vi "获取需发送的数据表.vi"(8 "error in (no error)":errorcluster) -> (0 "error out":errorcluster, 3 "tables":string[](array[string]))   [LabVIEW 2016, in "数据传输系统-03.lvlib"]
uses:
  <vilib>/Utility/sysdir.llb/System Directory Type.ctl
  <vilib>/addons/database/Connection.llb/DB Tools Open Connec (String).vi
  <vilib>/addons/database/NI_Database_API.lvlib
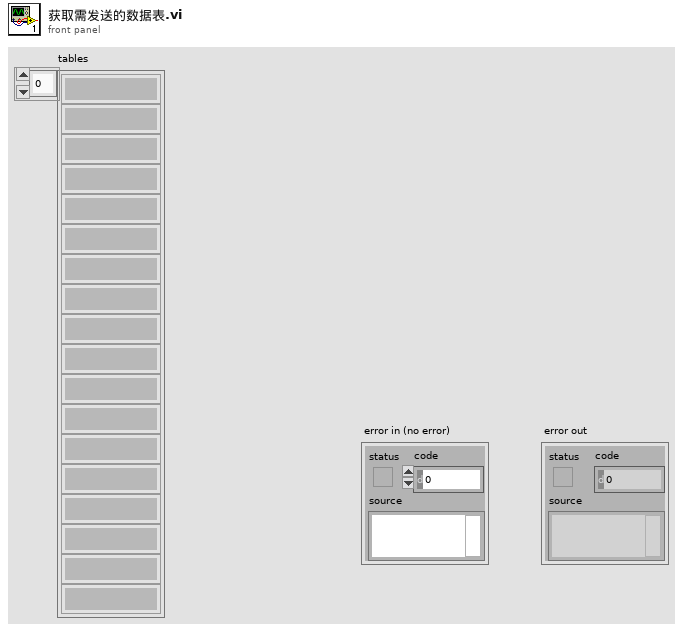
[diagram p1: front panel]
types:
  T1 = typedef "System Directory Type.ctl" = i32
  T2 = typedef "NI_Database_API.lvlib/Conn ObjectReference.ctl" = refnum<k1>
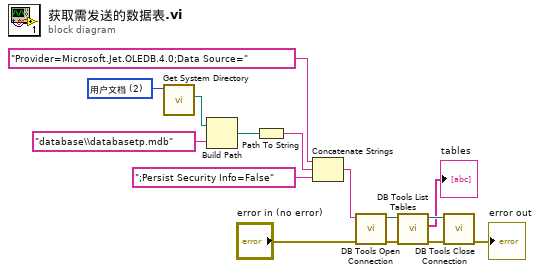
[diagram p0: block diagram]
diagram:
  w15 = T1 2 items=["用户目录"=0, "用户桌面"=1, "用户文档"=2, "用户应用程序数据"=3, "用户设置"=4, "用户临时目录"=5, "公共文档"=6, "公共应用程序数据"=7, "公共设置"=8, "公共缓存"=13, "系统核心库"=9, "系统安装库"=10, "应用程序文件"=11, "启动盘根目录"=12] ("system directory type")
  n1 = call <vilib>:"Get System Directory.vi"("system directory type"=w15) -> ("system directory"=w13:path)  [unwired: 10 in]
  n2 = Build Path(base path=w13, name or relative path="database\\databasetp.mdb" ("condition")) -> (appended path=w12:path)
  n3 = Path To String(path=w12) -> (string=w11:string)
  n4 = Concatenate Strings("Provider=Microsoft.Jet.OLEDB.4.0;Data Source=" ("condition"), w11, ";Persist Security Info=False" ("condition")) -> (w9:string)
  n5 = call-poly <vilib>:"DB Tools Open Connection.vi"("error in (no error)"="error in (no error)", "connection information"=w9) -> ("error out"=w6:errorcluster, "connection reference"=w7:T2)  [unwired: 6 in]
  n6 = call <vilib>:"DB Tools List Tables.vi"("error in (no error)"=w6, "connection reference"=w7) -> ("error out"=w4:errorcluster, "tables"=→"tables":string[], "connection reference out"=w5:T2)  [unwired: 3 in]
  n7 = call <vilib>:"DB Tools Close Connection.vi"("error in (no error)"=w4, "connection reference"=w5) -> ("error out"=→"error out":errorcluster)  [unwired: 5 in]
